vi "Init.vi"(8 "error in (no error)":errorcluster, 11 "reference in":refnum<class "Medulla_ATE.lvclass">) -> (0 "error out":errorcluster, 3 "reference out":refnum<class "Medulla_ATE.lvclass">)   [LabVIEW 2022 SP3, in "Medulla_ATE.lvlib" / "Medulla_ATE.lvclass"]
uses:
  Medulla_ATE.lvclass
  Components/ViPER.lvlibp/ViPER.lvclass
  C:/Projects/Medulla/ViPER/Examples/Flux_Capacitor_Tester/Components/ViPER.lvlibp/ViPER.lvclass
  Components/Test_Base.lvlibp/Test_Base.lvclass
  Components/DUT_Handler_Base.lvlibp/DUT_Handler_Base.lvclass
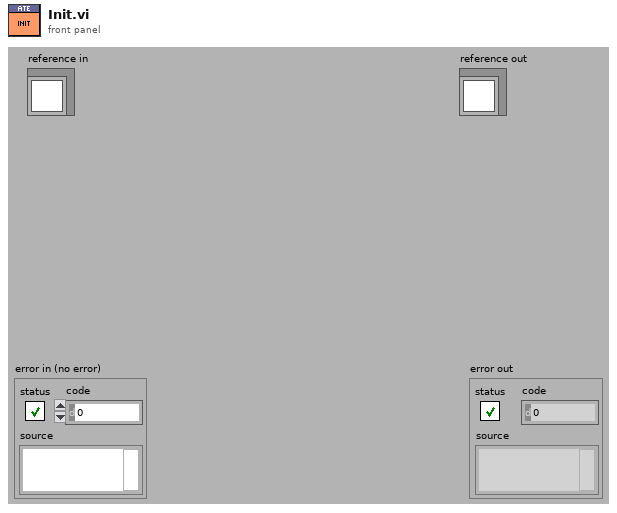
[diagram p1: front panel]
types:
  T1 = typedef "Medulla_ATE.lvlib/Medulla_ATE.lvclass/ObjectAttributes.ctl" = cluster{"Config":T2, "DUT_Handler":refnum<class "DUT_Handler_Base.lvclass">, "MES":refnum<class "MES_Base.lvclass">, "TestView":refnum<class "TestView_Base.lvclass">, "TestClass":refnum<class "Test_Base.lvclass">}
  T2 = typedef "Medulla_ATE.lvlib/Medulla_ATE.lvclass/Config.ctl" = cluster{"ForceStart":bool, "ForceAbort":bool}
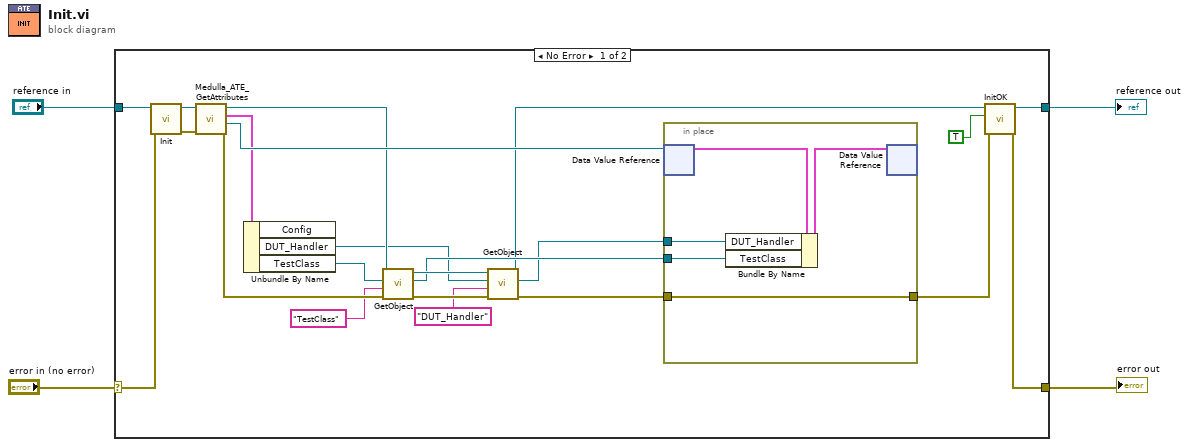
[diagram p0: block diagram]
diagram:
  n1 = case shown="No Error" "error in (no error)" {
    selector: "error in (no error)" -> [w25 w33]
    tunnel: [w18 w33] -> w3
    tunnel: [w21 w32] -> w1
    tunnel: "reference in" -> [w26 w32]
    frame No Error {
      n2 = call-parent "Init.vi"("error in (no error)"=w25, "reference in"=w26) -> ("error out"=w23:errorcluster, "reference out"=w24:refnum<class "Medulla_ATE.lvclass">)  [unwired: 8 in]
      n3 = call "Medulla_ATE_GetAttributes.vi"("error in (no error)"=w23, "reference in"=w24) -> ("error out"=w17:errorcluster, "DataRef"=w22:refnum<data-value>, "Data"=w15:T1, "reference out"=w16:refnum<class "Medulla_ATE.lvclass">)  [unwired: 6 in]
      n4 = Unbundle By Name(w15) -> ("DUT_Handler"=w8:refnum<class "DUT_Handler_Base.lvclass">, "TestClass"=w14:refnum<class "Test_Base.lvclass">)  [unwired: 1 out]
      n5 = call "GetObject.vi"("error in (no error)"=w17, "Object Name"="TestClass", "Class type"=w14, "reference in"=w16) -> ("error out"=w12:errorcluster, "Object out"=w9:refnum<class "Test_Base.lvclass">, "reference out"=w10:refnum<class "Medulla_ATE.lvclass">)  [unwired: 5 in]
      n6 = call "GetObject.vi"("error in (no error)"=w12, "Object Name"="DUT_Handler", "Class type"=w8, "reference in"=w10) -> ("error out"=w11:errorcluster, "Object out"=w6:refnum<class "DUT_Handler_Base.lvclass">, "reference out"=w5:refnum<class "Medulla_ATE.lvclass">)  [unwired: 5 in]
      n7 = in-place {
        in-place-border: w11 -> [w31]
        in-place-border: [w31] -> w19
        in-place-border: w9 -> [w28]
        in-place-border: w6 -> [w27]
        n8 = in-place-dvr #1(w22) -> (w30:T1)  [unwired: 1 out]
        n9 = Bundle By Name(cluster=w30, "DUT_Handler"=w27, "TestClass"=w28) -> (w29:T1)
        n10 = in-place-dvr #1(w29) -> ()  [unwired: 2 out]
      }
      n11 = call "InitOK.vi"("error in (no error)"=w19, "Init OK?"=TRUE, "reference in"=w5) -> ("error out"=w18:errorcluster, "reference out"=w21:refnum<class "Medulla_ATE.lvclass">)  [unwired: 7 in]
    }
    frame Error {
    }
  }
  "error out" <- w3
  "reference out" <- w1
